vi "rs3 post process4.vi"(0 "Depth Input":dbl[][](graph), 1 "Color input":u8[](array[numeric]), 2 "hole fill algo":i32(ring)=1 items=["filling with left pixel", "filling with biggest of nearest pixels", "filling with smallest of nearest pixels"], 3 "Temporal Credible table":u8[](array[numeric]), 4 "Algo step":enum16{"Start", "Continue", "End", "Do Nothing"}(ring)=enum."Continue", 5 "ID":i32, 6 "downsample  parameters":T4={"focal length (pixels)"=961.0, "baseline, mm"=0.015000001, "z_units"=0.001, "Y height"=720, "X width"=1280, "Scale"=3, "Color format"=enum."RGB internal (RGB)"} {"Scale" min=1 max=8}, 7 "Time average parameters":T3={"alphaT"=0.4, "deltaDispT(1/32 disp)"=10.0}, 8 "Temporal persistence \nHole-filling":enum16{"Custom", "Default", "Max holefilling"}(ring)=enum."Default", 9 "Spatial Filter":bool=TRUE, 10 "Time Filter":bool=TRUE, 11 "Holefill":bool, 12 "Spatial filter parameters":T2={"alphaXY"=0.6, "deltaDispXY (1/32 disp)"=10.0, "iterations"=2} {"iterations" min=1 max=8; "deltaDispXY (1/32 disp)" min=0.001 max=65000; "alphaXY" min=0.001 max=1}, 17 "transpose":bool) -> (13 "Processing time":T1={"downsample time, "=5, "temporal filter time"=0, "Spatial filter time"=0, "Back to depth time"=0, "Holefill time "=0}, 14 "Depth Output":sgl[][](graph), 15 "Color output":u8[](array[numeric]), 18 "output width":i32=428, 19 "output height":i32=240)   [LabVIEW 2017, in "libRealSense3.lvlib"]
uses:
  <vilib>/addons/RealSense/libRealSense3.lvlib
  <vilib>/addons/RealSense/realsense2ex.dll
panel:
  out "error out":errorcluster
  out "Return":u8=1
  # "RS3 Post Process"
  # "(C) Intel Corp. 2017,  AGJ"
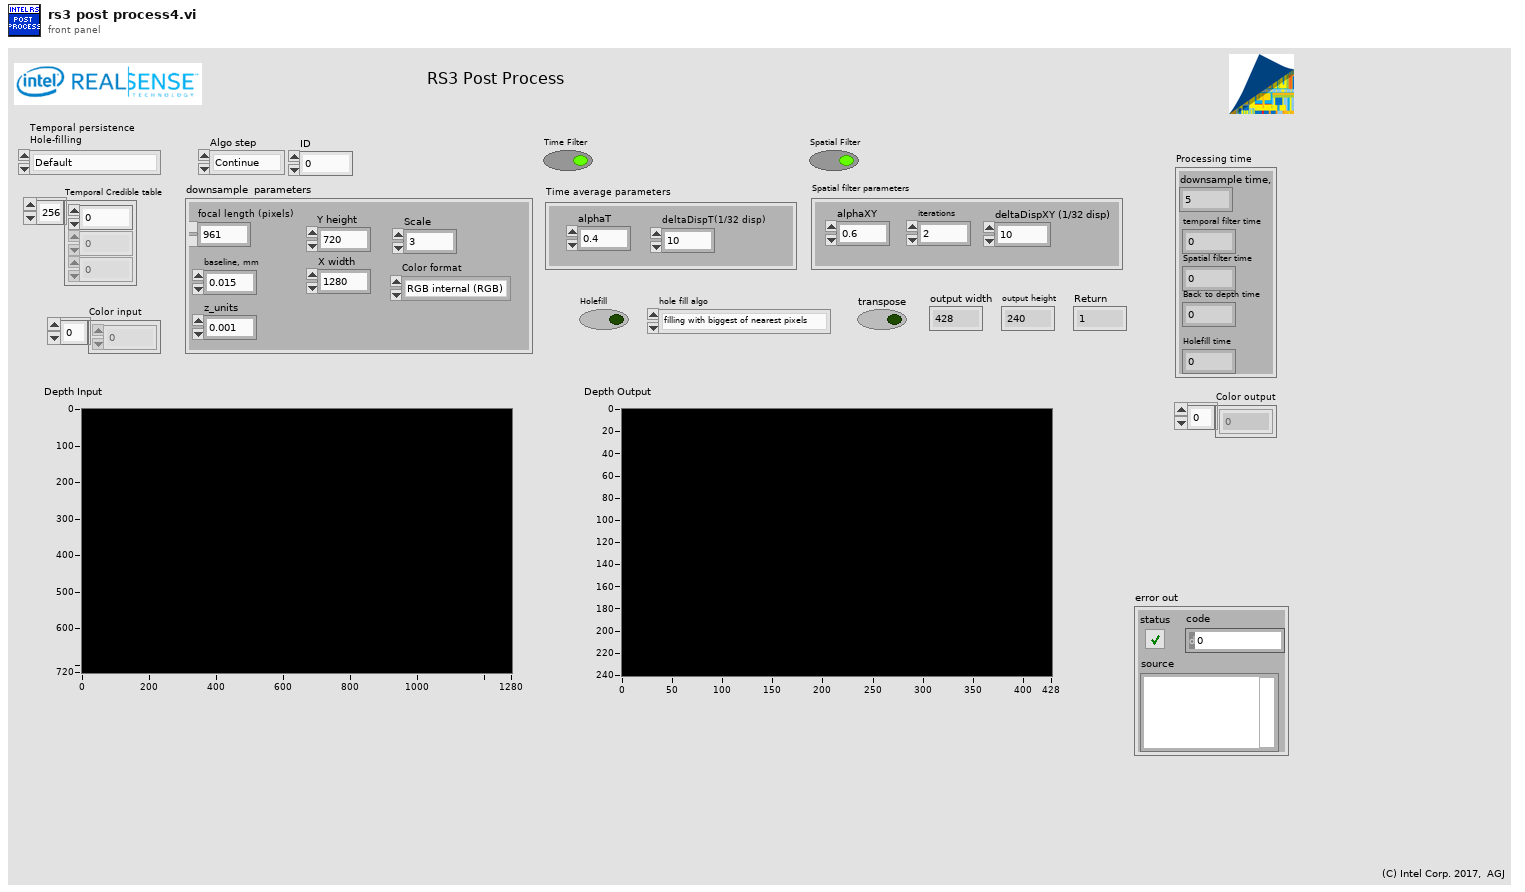
[diagram p1: front panel]
types:
  T1 = cluster{"downsample time, ":u32, "temporal filter time":u32, "Spatial filter time":u32, "Back to depth time":u32, "Holefill time ":u32}
  T2 = cluster{"alphaXY":sgl, "deltaDispXY (1/32 disp)":sgl, "iterations":i32}
  T3 = cluster{"alphaT":sgl, "deltaDispT(1/32 disp)":sgl}
  T4 = cluster{"focal length (pixels)":sgl, "baseline, mm":sgl, "z_units":sgl, "Y height":i32, "X width":i32, "Scale":i32, "Color format":enum16{"Monochrome", "RGB internal (RGB)"}}
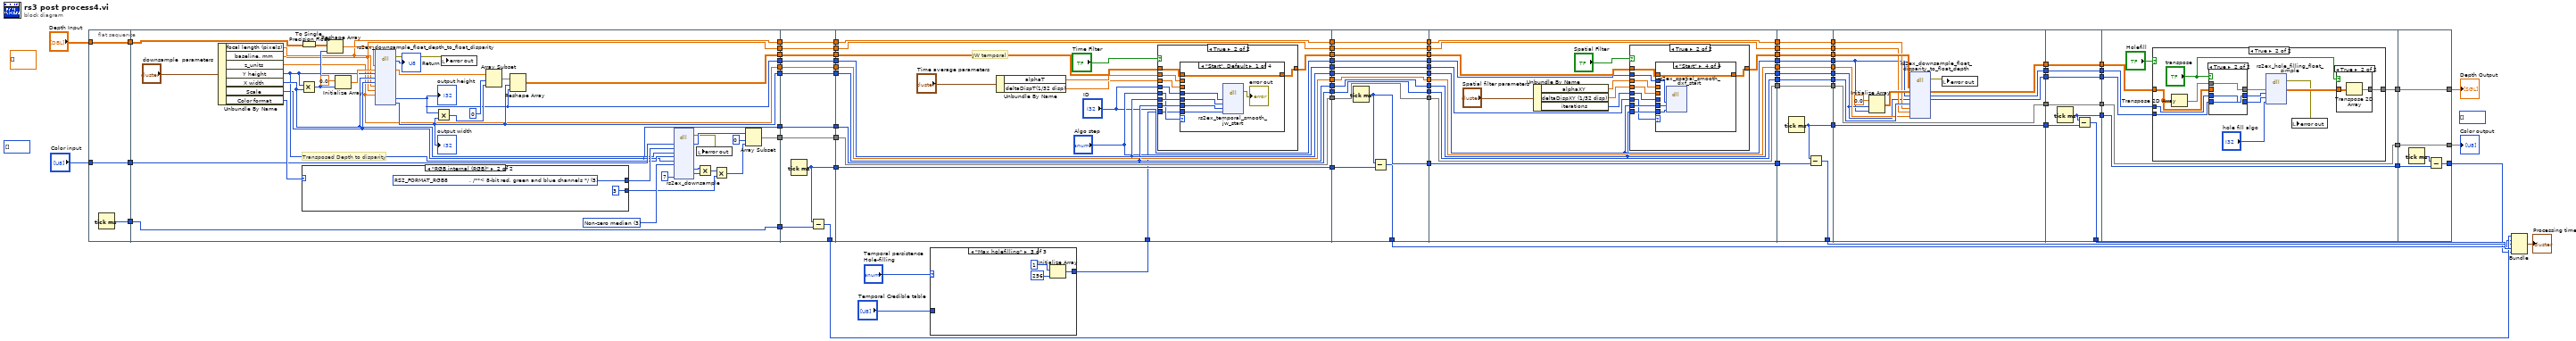
[diagram p0: block diagram]
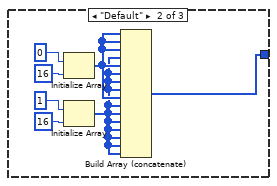
[diagram p3: hidden frame]
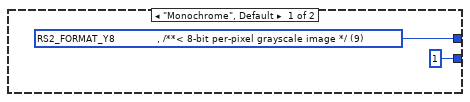
[diagram p4: hidden frame]
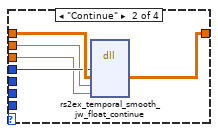
[diagram p6: hidden frame]
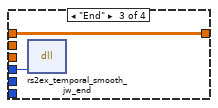
[diagram p7: hidden frame]
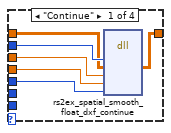
[diagram p10: hidden frame]
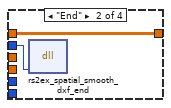
[diagram p11: hidden frame]
diagram:
  (unwired) u8[] []
  (unwired) u8[] [] ("Color input")
  (unwired) dbl[][] [] ("Depth Input")
  n1 = flat-sequence {
    tunnel: "Depth Input" -> [w89]
    tunnel: "Color input" -> [w90]
    tunnel: [w90] -> w87
    tunnel: [w89] -> w86
    tunnel: [w88] -> w66
    tunnel: w87 -> [w106]
    tunnel: w86 -> [w105]
    tunnel: [w104] -> w85
    tunnel: [w103] -> w84
    tunnel: [w97] -> w81
    tunnel: [w98] -> w79
    tunnel: [w100] -> w67
    tunnel: w66 -> [w100]
    tunnel: [w96] -> w50
    tunnel: [w95] -> w49
    tunnel: [w94] -> w38
    tunnel: [w93] -> w37
    tunnel: w85 -> [w142]
    tunnel: w84 -> [w141]
    tunnel: [w142] -> w83
    tunnel: [w141] -> w82
    tunnel: w81 -> [w140]
    tunnel: [w140] -> w80
    tunnel: w79 -> [w139]
    tunnel: [w139] -> w78
    tunnel: w67 -> [w138]
    tunnel: [w137] -> w65
    tunnel: [w136] -> w51
    tunnel: w50 -> [w136]
    tunnel: w49 -> [w135]
    tunnel: [w135] -> w48
    tunnel: [w134] -> w39
    tunnel: w38 -> [w134]
    tunnel: w37 -> [w133]
    tunnel: [w133] -> w36
    tunnel: [w132] -> w23
    tunnel: w83 -> [w155]
    tunnel: w82 -> [w159]
    tunnel: w80 -> [w153]
    tunnel: w78 -> [w152]
    tunnel: [w154] -> w77
    tunnel: [w159] -> w76
    tunnel: [w153] -> w73
    tunnel: [w152] -> w70
    tunnel: w65 -> [w151]
    tunnel: [w151] -> w64
    tunnel: [w150] -> w52
    tunnel: w51 -> [w150]
    tunnel: w48 -> [w149]
    tunnel: [w149] -> w47
    tunnel: [w148] -> w40
    tunnel: w39 -> [w148]
    tunnel: w36 -> [w147]
    tunnel: [w147] -> w35
    tunnel: ["Algo step"] -> w27
    tunnel: ["ID"] -> w18
    tunnel: w5 -> [w143]
    tunnel: w77 -> [w196]
    tunnel: w76 -> [w195]
    tunnel: [w196] -> w75
    tunnel: [w195] -> w74
    tunnel: w73 -> [w194]
    tunnel: [w194] -> w72
    tunnel: [w193] -> w71
    tunnel: w70 -> [w193]
    tunnel: w64 -> [w192]
    tunnel: [w191] -> w63
    tunnel: [w190] -> w53
    tunnel: w52 -> [w190]
    tunnel: w47 -> [w189]
    tunnel: [w189] -> w46
    tunnel: [w188] -> w41
    tunnel: w40 -> [w188]
    tunnel: w35 -> [w187]
    tunnel: [w187] -> w34
    tunnel: w27 -> [w186]
    tunnel: [w186] -> w26
    tunnel: [w185] -> w22
    tunnel: [w184] -> w19
    tunnel: w18 -> [w184]
    tunnel: w75 -> [w208]
    tunnel: w74 -> [w213]
    tunnel: w72 -> [w205]
    tunnel: w71 -> [w204]
    tunnel: [w207] -> w69
    tunnel: [w213] -> w68
    tunnel: w63 -> [w206]
    tunnel: [w206] -> w62
    tunnel: [w205] -> w58
    tunnel: [w204] -> w56
    tunnel: [w203] -> w54
    tunnel: w53 -> [w203]
    tunnel: w46 -> [w202]
    tunnel: [w202] -> w45
    tunnel: [w201] -> w42
    tunnel: w41 -> [w201]
    tunnel: w34 -> [w200]
    tunnel: [w200] -> w33
    tunnel: w26 -> [w199]
    tunnel: w19 -> [w198]
    tunnel: w69 -> [w247]
    tunnel: w68 -> [w246]
    tunnel: w62 -> [w245]
    tunnel: [w247] -> w61
    tunnel: [w246] -> w60
    tunnel: [w244] -> w59
    tunnel: w58 -> [w244]
    tunnel: [w243] -> w57
    tunnel: w56 -> [w243]
    tunnel: [w242] -> w55
    tunnel: w54 -> [w242]
    tunnel: w45 -> [w241]
    tunnel: [w241] -> w44
    tunnel: [w240] -> w43
    tunnel: w42 -> [w240]
    tunnel: w33 -> [w239]
    tunnel: [w239] -> w32
    tunnel: [w238] -> w28
    tunnel: [w237] -> w21
    tunnel: w61 -> [w261]
    tunnel: w60 -> [w262]
    tunnel: w59 -> [w253]
    tunnel: w57 -> [w254]
    tunnel: w55 -> [w258]
    tunnel: w44 -> [w257]
    tunnel: w43 -> [w256]
    tunnel: w32 -> [w255]
    tunnel: [w249] -> w31
    tunnel: [w262] -> w30
    tunnel: [w252] -> w29
    tunnel: w28 -> [w252]
    tunnel: [w251] -> w12
    tunnel: [w250] -> w10
    tunnel: w31 -> [w269]
    tunnel: w30 -> [w268]
    tunnel: w29 -> [w267]
    tunnel: [w266] -> w24
    tunnel: [w269] -> w17
    tunnel: [w268] -> w16
    tunnel: [w265] -> w13
    tunnel: w12 -> [w265]
    tunnel: [w264] -> w11
    tunnel: w10 -> [w264]
    tunnel: [w263] -> w8
    tunnel: w17 -> [w275]
    tunnel: w16 -> [w276]
    tunnel: [w274] -> w15
    tunnel: [w276] -> w14
    tunnel: w13 -> [w272]
    tunnel: w11 -> [w271]
    tunnel: [w270] -> w9
    tunnel: w8 -> [w270]
    tunnel: [w302] -> w2
    tunnel: [w303] -> w25
    tunnel: w15 -> [w303]
    tunnel: w14 -> [w302]
    tunnel: w9 -> [w300]
    tunnel: [w299] -> w7
    frame #0 {
      n2 = Tick Count (ms)() -> (millisecond timer value=w88:u32)
    }
    frame #1 {
      w127 = u16 3 items=["Fixed Pick", "Random Pick", "Median", "Non-zero median", "non-zero mean", "thresh mean"] ("Downscale algo Depth")
      # "Transposed Depth to disparity"
      n3 = Unbundle By Name("downsample  parameters") -> ("focal length (pixels)"=w95:sgl, "baseline, mm"=w94:sgl, "z_units"=w93:sgl, "Y height"=w99:i32, "X width"=w101:i32, "Scale"=w96:i32, "Color format"=w109:enum16{"Monochrome", "RGB internal (RGB)"})
      n4 = Multiply(x=w99, y=w101) -> (x*y=w108:i32)
      n5 = To Single Precision Float(number=w105) -> (single precision float=w121:sgl[][])
      n6 = case shown="\"RGB internal (RGB)\"" w109 {
        tunnel: [w129 w131] -> w120
        tunnel: [1 ("y") 3 ("y")] -> w112
        frame "Monochrome", Default {
          w129 = u16 9 items=["    RS2_FORMAT_ANY             , /**< When passed to enable stream, librealsense will try to provide best suited format */", "    RS2_FORMAT_Z16             , /**< 16-bit linear depth values. The depth is meters is equal to depth scale * pixel value. */", "    RS2_FORMAT_DISPARITY16     , /**< 16-bit linear disparity values. The depth in meters is equal to depth scale / pixel value. */", "    RS2_FORMAT_XYZ32F          , /**< 32-bit floating point 3D coordinates. */", "    RS2_FORMAT_YUYV            , /**< Standard YUV pixel format as described in https://en.wikipedia.org/wiki/YUV */", "    RS2_FORMAT_RGB8            , /**< 8-bit red, green and blue channels */", "    RS2_FORMAT_BGR8            , /**< 8-bit blue, green, and red channels -- suitable for OpenCV */", "    RS2_FORMAT_RGBA8           , /**< 8-bit red, green and blue channels + constant alpha channel equal to FF */", "    RS2_FORMAT_BGRA8           , /**< 8-bit blue, green, and red channels + constant alpha channel equal to FF */", "    RS2_FORMAT_Y8              , /**< 8-bit per-pixel grayscale image */", "    RS2_FORMAT_Y16             , /**< 16-bit per-pixel grayscale image */", "    RS2_FORMAT_RAW10           , /**< Four 10-bit luminance values encoded into a 5-byte macropixel */", "    RS2_FORMAT_RAW16           , /**< 16-bit raw image */", "    RS2_FORMAT_RAW8            , /**< 8-bit raw image */", "    RS2_FORMAT_UYVY            , /**< Similar to the standard YUYV pixel format, but packed in a different order */", "    RS2_FORMAT_MOTION_RAW      , /**< Raw data from the motion sensor */", "    RS2_FORMAT_MOTION_XYZ32F   , /**< Motion data packed as 3 32-bit float values, for X, Y, and Z axis */", "    RS2_FORMAT_GPIO_RAW        , /**< Raw data from the external sensors hooked to one of the GPIO's */", "    RS2_FORMAT_COUNT             /**< Number of enumeration values. Not a valid input: intended to be used in for-loops. */"] ("RS Format")
        }
        frame "RGB internal (RGB)" {
          w131 = u16 5 items=["    RS2_FORMAT_ANY             , /**< When passed to enable stream, librealsense will try to provide best suited format */", "    RS2_FORMAT_Z16             , /**< 16-bit linear depth values. The depth is meters is equal to depth scale * pixel value. */", "    RS2_FORMAT_DISPARITY16     , /**< 16-bit linear disparity values. The depth in meters is equal to depth scale / pixel value. */", "    RS2_FORMAT_XYZ32F          , /**< 32-bit floating point 3D coordinates. */", "    RS2_FORMAT_YUYV            , /**< Standard YUV pixel format as described in https://en.wikipedia.org/wiki/YUV */", "    RS2_FORMAT_RGB8            , /**< 8-bit red, green and blue channels */", "    RS2_FORMAT_BGR8            , /**< 8-bit blue, green, and red channels -- suitable for OpenCV */", "    RS2_FORMAT_RGBA8           , /**< 8-bit red, green and blue channels + constant alpha channel equal to FF */", "    RS2_FORMAT_BGRA8           , /**< 8-bit blue, green, and red channels + constant alpha channel equal to FF */", "    RS2_FORMAT_Y8              , /**< 8-bit per-pixel grayscale image */", "    RS2_FORMAT_Y16             , /**< 16-bit per-pixel grayscale image */", "    RS2_FORMAT_RAW10           , /**< Four 10-bit luminance values encoded into a 5-byte macropixel */", "    RS2_FORMAT_RAW16           , /**< 16-bit raw image */", "    RS2_FORMAT_RAW8            , /**< 8-bit raw image */", "    RS2_FORMAT_UYVY            , /**< Similar to the standard YUYV pixel format, but packed in a different order */", "    RS2_FORMAT_MOTION_RAW      , /**< Raw data from the motion sensor */", "    RS2_FORMAT_MOTION_XYZ32F   , /**< Motion data packed as 3 32-bit float values, for X, Y, and Z axis */", "    RS2_FORMAT_GPIO_RAW        , /**< Raw data from the external sensors hooked to one of the GPIO's */", "    RS2_FORMAT_COUNT             /**< Number of enumeration values. Not a valid input: intended to be used in for-loops. */"] ("RS Format")
        }
      }
      n7 = Reshape Array(w121, w108) -> (w122:sgl[])
      n8 = Initialize Array(sgl 0.0 ("element"), w108) -> (w123:sgl[])
      n9 = dll-call lib="C:/Users/agrunnet/Documents/LabVIEW libRealSense5/libRealSense5/realsense2ex.dll" fn="rs2ex_downsample_float_depth_to_float_disparity"("depth frame array"=w122, "disparity map"=w123, "width"=w99, "height"=w101, "scale"=w96, "focal length (pixels)"=w95, "baseline"=w94, "z_units"=w93) -> (error out=w91:errorcluster, "return"=→"Return":u8, "disparity map"=w110:sgl[], "output width"=w97:i32, "output height"=w98:i32)  [unwired: 12 in, 1 out]
      "output height" <- w97
      "output width" <- w98
      n10 = Multiply(x=w97, y=w98) -> (x*y=w119:i32)
      n11 = local write "error out"(w91) -> ()
      n12 = Array Subset(array=w110, index=0, length=w119) -> (w118:sgl[])
      n13 = Reshape Array(w118, w98, w97) -> (w104:sgl[][])
      n14 = dll-call lib="C:/Users/agrunnet/Documents/LabVIEW libRealSense5/libRealSense5/realsense2ex.dll" fn="rs2ex_downsample"("frame data pointer"=w106, "format"=w120, "width"=w101, "height"=w99, "scale"=w96, "downscale algo"=w127, "param"=7) -> (error out=w92:errorcluster, "frame data pointer"=w113:u8[], "output width"=w117:i32, "output height"=w116:i32)  [unwired: 12 in, 1 out]
      n15 = local write "error out"(w92) -> ()
      n16 = Multiply(x=w117, y=w116) -> (x*y=w115:i32)
      n17 = Multiply(x=w115, y=w112) -> (x*y=w114:i32)
      n18 = Array Subset(array=w113, index=0, length=w114) -> (w103:u8[])
    }
    frame #2 {
      n19 = Tick Count (ms)() -> (millisecond timer value=w137:u32)
      n20 = Subtract(x=w137, y=w138) -> (x-y=w132:u32)
    }
    frame #3 {
      # "JW temporal"
      n21 = Unbundle By Name("Time average parameters") -> ("alphaT"=w157:sgl, "deltaDispT(1/32 disp)"=w156:sgl)
      n22 = case shown="True" "Time Filter" {
        tunnel: w157 -> [_ w169]
        tunnel: w156 -> [_ w168]
        tunnel: w155 -> [w160 w167]
        tunnel: [w160 w166] -> w154
        tunnel: w153 -> [_ w165]
        tunnel: w152 -> [_ w164]
        tunnel: "Algo step" -> [_ w163]
        tunnel: "ID" -> [_ w162]
        tunnel: w143 -> [_ w161]
        frame False {
        }
        frame True {
          n23 = case shown="\"Start\", Default" w163 {
            tunnel: w167 -> [w175 w179 w182 w183]
            tunnel: [w175 w180 w182 w183] -> w166
            tunnel: w162 -> [w174 w178 w181 _]
            tunnel: w169 -> [_ w177 _ _]
            tunnel: w168 -> [_ w176 _ _]
            tunnel: w165 -> [w173 _ _ _]
            tunnel: w164 -> [w172 _ _ _]
            tunnel: w161 -> [w170 _ _ _]
            frame "Start", Default {
              n24 = dll-call lib="C:/Users/agrunnet/Documents/LabVIEW libRealSense5/libRealSense5/realsense2ex.dll" fn="rs2ex_temporal_smooth_jw_start"("ID"=w174, "width"=w173, "height"=w172, "Credible table"=w170) -> (error out=→"error out":errorcluster)  [unwired: 8 in, 1 out]
            }
            frame "Continue" {
              n25 = dll-call lib="C:/Users/agrunnet/Documents/LabVIEW libRealSense5/libRealSense5/realsense2ex.dll" fn="rs2ex_temporal_smooth_jw_float_continue"("ID"=w178, "disparity 2D array"=w179, "alphaT"=w177, "deltaDispT"=w176) -> ("disparity 2D array"=w180:sgl[][])  [unwired: 7 in, 2 out]
            }
            frame "End" {
              n26 = dll-call lib="C:/Users/agrunnet/Documents/LabVIEW libRealSense5/libRealSense5/realsense2ex.dll" fn="rs2ex_temporal_smooth_jw_end"("ID"=w181) -> ()  [unwired: 5 in, 2 out]
            }
            frame "Do Nothing" {
            }
          }
        }
      }
    }
    frame #4 {
      n27 = Tick Count (ms)() -> (millisecond timer value=w191:u32)
      n28 = Subtract(x=w191, y=w192) -> (x-y=w185:u32)
    }
    frame #5 {
      n29 = Unbundle By Name("Spatial filter parameters") -> ("alphaXY"=w211:sgl, "deltaDispXY (1/32 disp)"=w210:sgl, "iterations"=w209:i32)
      n30 = case shown="True" "Spatial Filter" {
        tunnel: w211 -> [_ w223]
        tunnel: w210 -> [_ w222]
        tunnel: w209 -> [_ w221]
        tunnel: w208 -> [w214 w220]
        tunnel: [w214 w219] -> w207
        tunnel: w205 -> [_ w218]
        tunnel: w204 -> [_ w217]
        tunnel: w199 -> [_ w216]
        tunnel: w198 -> [_ w215]
        frame False {
        }
        frame True {
          n31 = case shown="\"Start\"" w216 {
            tunnel: w218 -> [_ _ _ w236]
            tunnel: w217 -> [_ _ _ w235]
            tunnel: w215 -> [w229 w231 _ w234]
            tunnel: w223 -> [w228 _ _ _]
            tunnel: w222 -> [w227 _ _ _]
            tunnel: w221 -> [w226 _ _ _]
            tunnel: w220 -> [w225 w230 w232 w233]
            tunnel: [w224 w230 w232 w233] -> w219
            frame "Continue" {
              n32 = dll-call lib="C:/Users/agrunnet/Documents/LabVIEW libRealSense5/libRealSense5/realsense2ex.dll" fn="rs2ex_spatial_smooth_float_dxf_continue"("ID"=w229, "2D disparity array"=w225, "alpha"=w228, "delta"=w227, "iterations"=w226) -> ("2D disparity array"=w224:sgl[][])  [unwired: 8 in, 2 out]
            }
            frame "End" {
              n33 = dll-call lib="C:/Users/agrunnet/Documents/LabVIEW libRealSense5/libRealSense5/realsense2ex.dll" fn="rs2ex_spatial_smooth_dxf_end"("ID"=w231) -> ()  [unwired: 5 in, 2 out]
            }
            frame "Do Nothing" {
            }
            frame "Start" {
              n34 = dll-call lib="C:/Users/agrunnet/Documents/LabVIEW libRealSense5/libRealSense5/realsense2ex.dll" fn="rs2ex_spatial_smooth_dxf_start"("ID"=w234, "width"=w236, "height"=w235) -> ()  [unwired: 7 in, 2 out]
            }
          }
        }
      }
    }
    frame #6 {
      n35 = Tick Count (ms)() -> (millisecond timer value=w238:u32)
      n36 = Subtract(x=w238, y=w245) -> (x-y=w237:u32)
    }
    frame #7 {
      n37 = Initialize Array(sgl 0.0 ("element"), w254, w253) -> (w259:sgl[][])
      n38 = dll-call lib="C:/Users/agrunnet/Documents/LabVIEW libRealSense5/libRealSense5/realsense2ex.dll" fn="rs2ex_downsample_float_disparity_to_float_depth" label="rs2ex_downsample_float_disparity_to_depth"("disparity map input"=w261, "depth map output"=w259, "width"=w253, "height"=w254, "scale"=w258, "focal length (pixels)"=w257, "baseline"=w256, "z_unit"=w255) -> (error out=w248:errorcluster, "depth map output"=w249:sgl[][], "width"=w251:i32, "height"=w250:i32)  [unwired: 9 in, 1 out]
      n39 = local write "error out"(w248) -> ()
    }
    frame #8 {
      n40 = Tick Count (ms)() -> (millisecond timer value=w263:u32)
      n41 = Subtract(x=w263, y=w267) -> (x-y=w266:u32)
    }
    frame #9 {
      n42 = case shown="True" "Holefill" {
        tunnel: w275 -> [w277 w288]
        tunnel: [w277 w279] -> w274
        tunnel: w272 -> [_ w284]
        tunnel: w271 -> [_ w283]
        frame False {
        }
        frame True {
          n43 = Transpose 2D Array(2D array=w288) -> (transposed array=w286:sgl[][])
          n44 = case shown="True" "transpose" {
            tunnel: [w295 w298] -> w287
            tunnel: w288 -> [w295 _]
            tunnel: w286 -> [_ w298]
            tunnel: [w294 w297] -> w285
            tunnel: w284 -> [w294 w296]
            tunnel: w283 -> [w293 w297]
            tunnel: [w293 w296] -> w282
            frame False {
            }
            frame True {
            }
          }
          n45 = dll-call lib="C:/Users/agrunnet/Documents/LabVIEW libRealSense5/libRealSense5/realsense2ex.dll" fn="rs2ex_hole_filling_float_simple" label="rs2ex_simplehole filling"("depth map"=w287, "width"=w285, "height"=w282, "flag"="hole fill algo") -> (error out=w278:errorcluster, "depth map"=w280:sgl[][])  [unwired: 7 in, 1 out]
          n46 = local write "error out"(w278) -> ()
          n47 = case shown="True" "transpose" {
            tunnel: w280 -> [w290 w292]
            tunnel: [w290 w291] -> w279
            frame False {
            }
            frame True {
              n48 = Transpose 2D Array(2D array=w292) -> (transposed array=w291:sgl[][])
            }
          }
        }
      }
    }
    frame #10 {
      n49 = Tick Count (ms)() -> (millisecond timer value=w301:u32)
      n50 = Subtract(x=w301, y=w300) -> (x-y=w299:u32)
    }
  }
  n51 = case shown="\"Max holefilling\"" "Temporal persistence \nHole-filling" {
    tunnel: [w304 w305 w312] -> w5
    tunnel: "Temporal Credible table" -> [w304 _ _]
    frame "Custom", Default {
    }
    frame "Default" {
      n52 = Initialize Array(u8 0 ("element"), 16 ("dimension size")) -> (w307:u8[])
      n53 = Initialize Array(u8 1 ("element"), 16 ("dimension size")) -> (w306:u8[])
      n54 = Build Array (concatenate)(w307, w307, w307, w306, w307, w306, w306, w306, w307, w306, w306, w306, w306, w306, w306, w306) -> (w305:u8[])
    }
    frame "Max holefilling" {
      n55 = Initialize Array(u8 1 ("element"), 256 ("dimension size")) -> (w312:u8[])
    }
  }
  n56 = Bundle(w23, w22, w21, w24, w7) -> (→"Processing time":cluster{u32, u32, u32, u32, u32})  [unwired: 1 in]
  "Color output" <- w2
  "Depth Output" <- w25
